vi "CLD 4 Event Structure Timer Front Panel.vi"() -> ()   [LabVIEW 2014]
doc: "CLD-Zusatzaufgabe 4"
panel:
  out "Fehler (Ausgang)":T1
  in  "Fehler (Eingang)":T1
  out "Bit 4":bool
  out "Bit 3":bool
  out "Bit 2":bool
  out "Bit 1":bool
  out "Zeit ist verstrichen":bool
  out "Verstrichene Zeit":string
  in  "Autom. zurücksetzen":bool=TRUE
  in  "Zurücksetzen-Schaltfläche":bool
  in  "VI anhalten":bool
  in  "Zielzeit (s)":dbl=4.0
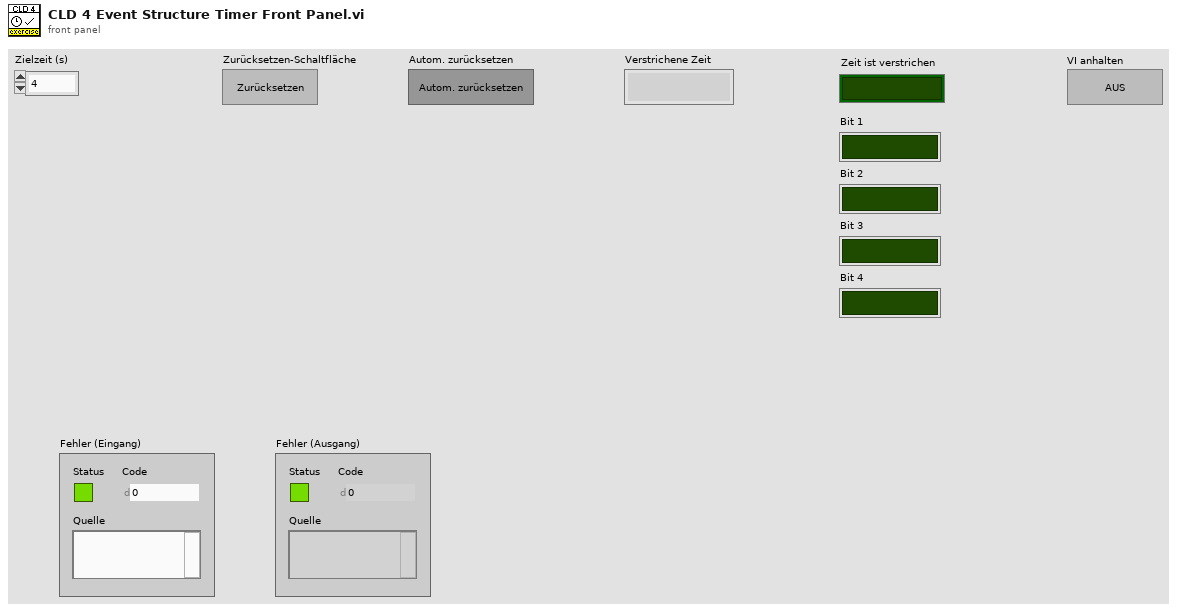
[diagram p1: front panel]
types:
  T1 = cluster{"Status":bool, "Code":i32, "Quelle":string}
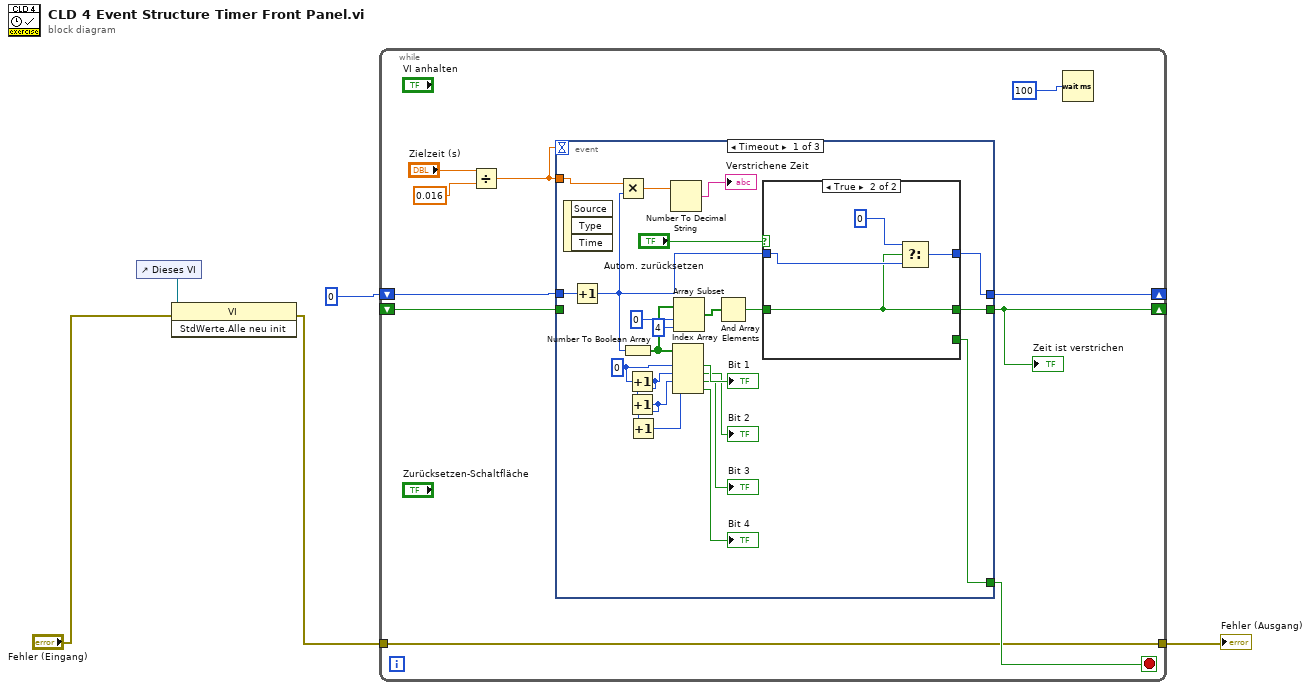
[diagram p0: block diagram]
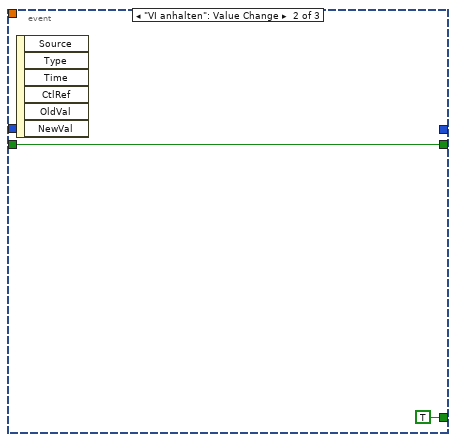
[diagram p3: hidden frame]
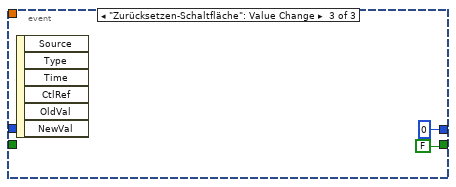
[diagram p4: hidden frame]
diagram:
  n1 = control-ref of="Dieses VI"() -> (w3:refnum<vi>)
  n2 = invoke class="VI" method="StdWerte.Alle neu init"(reference=w3, error in="Fehler (Eingang)") -> (error out=w1:errorcluster)  [unwired: 1 in, 2 out]
  n3 = while {
    shift-right: [w13] -> _
    shift-left: 0 -> [w12]
    shift-right: [w10] -> _
    shift-left: _ -> [w9]
    tunnel: w1 -> [w8]
    tunnel: [w8] -> w4
    stop <- w11 stop-if-true
    n4 = Divide(x="Zielzeit (s)", y=0.016) -> (x/y=w7:dbl)
    n5 = event shown="[0] Timeout" {
      selector: _ -> [_ _ _]
      dyn-events: _ -> [_ _ _]
      timeout: w7 -> [_ _ _]
      tunnel: [w27 _ 0] -> w13
      tunnel: w12 -> [w37 _ _]
      tunnel: [w20 w44 FALSE] -> w10
      tunnel: [w26 TRUE _] -> w11
      tunnel: w9 -> [_ w44 _]
      tunnel: w7 -> [w25 _ _]
      event Timeout {
        w36 = 0 ("Index")
        n6 = event-data() -> ()  [unwired: 1 in, 3 out]
        n7 = Increment(x=w37) -> (x+1=w24:i32)
        n8 = Multiply(x=w25, y=w24) -> (x*y=w23:dbl)
        n9 = Number To Boolean Array(number=w24) -> (Boolean array=w19:bool[])
        n10 = Increment(x=w36) -> (x+1=w35:i32)
        n11 = Increment(x=w35) -> (x+1=w33:i32)
        n12 = Increment(x=w33) -> (x+1=w34:i32)
        n13 = Number To Decimal String(number=w23) -> (decimal integer string=→"Verstrichene Zeit":string)  [unwired: 1 in]
        n14 = Index Array(array=w19, index #1=w36, index #2=w35, index #3=w33, index #4=w34) -> (element #1=→"Bit 1":bool, element #2=→"Bit 2":bool, element #3=→"Bit 3":bool, element #4=→"Bit 4":bool)
        n15 = Array Subset(array=w19, index=0 ("Index"), length=4 ("Länge")) -> (w16:bool[])
        n16 = And Array Elements(Boolean array=w16) -> (logical AND=w21:bool)
        n17 = case shown="True" "Autom. zurücksetzen" {
          tunnel: [w39 w42] -> w27
          tunnel: [w38 _] -> w26
          tunnel: w24 -> [w39 w43]
          tunnel: w21 -> [w38 w40]
          tunnel: [w38 w40] -> w20
          frame False {
          }
          frame True {
            n18 = Select(t=0, s=w40, f=w43) -> (s? t:f=w42:i32)
          }
        }
      }
      event "VI anhalten": Value Change {
        n19 = event-data() -> ()  [unwired: 1 in, 6 out]
      }
      event "Zurücksetzen-Schaltfläche": Value Change {
        n20 = event-data() -> ()  [unwired: 1 in, 6 out]
      }
    }
    "Zeit ist verstrichen" <- w10
    n21 = Wait (ms)(milliseconds to wait=u32 100) -> ()  [unwired: 1 out]
  }
  "Fehler (Ausgang)" <- w4
